vi "Readexcel.vi"(10 "start (0, 0)":cluster{"start row":i32, "start column":i32}={"start row"=2, "start column"=1}) -> (3 "Excel设置码":string)   [LabVIEW 2019]
uses:
  <vilib>/Utility/NIReport.llb/Report Type.ctl
  <vilib>/Utility/sysdir.llb/System Directory Type.ctl
  <vilib>/addons/_office/excel.llb/Excel Get Data (str).vi
  <vilib>/Utility/NIReport.llb/NI_report.lvclass
  <vilib>/addons/_office/NI_ReportGenerationToolkit.lvlib
  <vilib>/Utility/NIReport.llb/NI_ReportGenerationCore.lvlib
  <vilib>/Utility/NIReport.llb/Excel/NI_Excel.lvclass
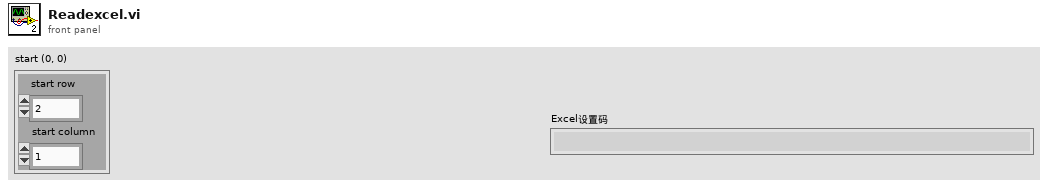
[diagram p1: front panel]
types:
  T1 = typedef "System Directory Type.ctl" = i32
  T2 = typedef "NI_ReportGenerationCore.lvlib/Report Type.ctl" = enum16{"HTML", "Word", "Excel"}
  T3 = enum16{"maximized", "minimized", "normal", "no change"}
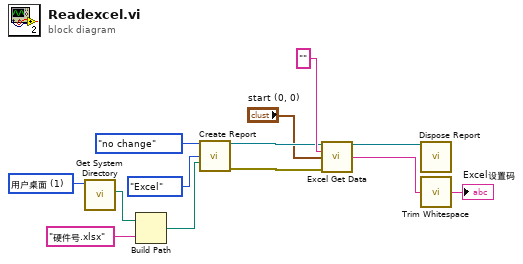
[diagram p0: block diagram]
diagram:
  w7 = T1 1 items=["用户目录"=0, "用户桌面"=1, "用户文档"=2, "用户应用程序数据"=3, "用户设置"=4, "用户临时目录"=5, "公共文档"=6, "公共应用程序数据"=7, "公共设置"=8, "公共缓存"=13, "系统核心库"=9, "系统安装库"=10, "应用程序文件"=11, "启动盘根目录"=12] ("system directory type")
  n1 = call <vilib>:"Get System Directory.vi"("system directory type"=w7) -> ("system directory"=w6:path)  [unwired: 10 in]
  n2 = Build Path(base path=w6, name or relative path="硬件号.xlsx" ("名称或相对路径")) -> (appended path=w4:path)
  n3 = call <vilib>:"Create Report.vi"("window state (normal)"=T3."no change", "report type"=Report_Type."Excel", "template (empty)"=w4) -> ("report out"=w12:refnum<class "NI_report.lvclass">, "error out"=w8:errorcluster)  [unwired: 11 in]
  n4 = call-poly <vilib>:"Excel Get Data.vi"("report in"=w12, "data type"="", "start (0, 0)"="start (0, 0)", "error in (no error)"=w8) -> ("report out"=w2:refnum<class "NI_report.lvclass">, "data"=w9:string)  [unwired: 9 in, 1 out]
  n5 = call-dynamic "Dispose Report.vi"("report in"=w2) -> ()  [unwired: 14 in, 1 out]
  n6 = call <vilib>:"Trim Whitespace.vi"("string"=w9) -> ("trimmed string"=→"Excel设置码":string)  [unwired: 1 in]
